vi "Init.vi"(8 "error in (no error)":errorcluster, 11 "Messages Actor in":refnum<class "Messages Actor.lvclass">) -> (0 "error out":errorcluster, 3 "Messages Actor out":refnum<class "Messages Actor.lvclass">)   [LabVIEW 2020, in "Messages Actor.lvlib" / "Messages Actor.lvclass"]
uses:
  Messages Actor.lvclass
  Messages Actor.lvclass/Messages Actor.ctl
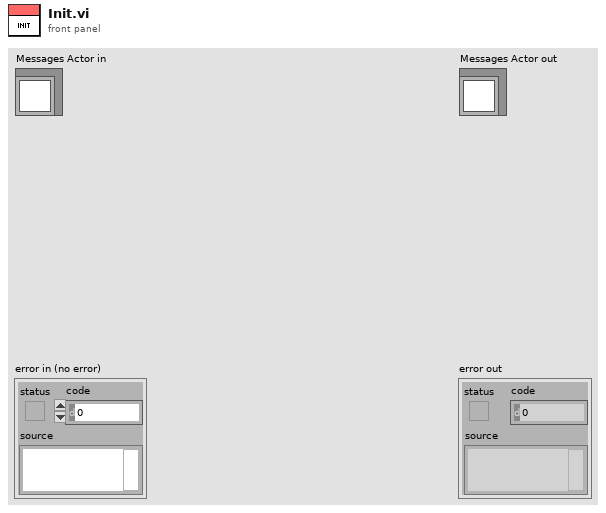
[diagram p1: front panel]
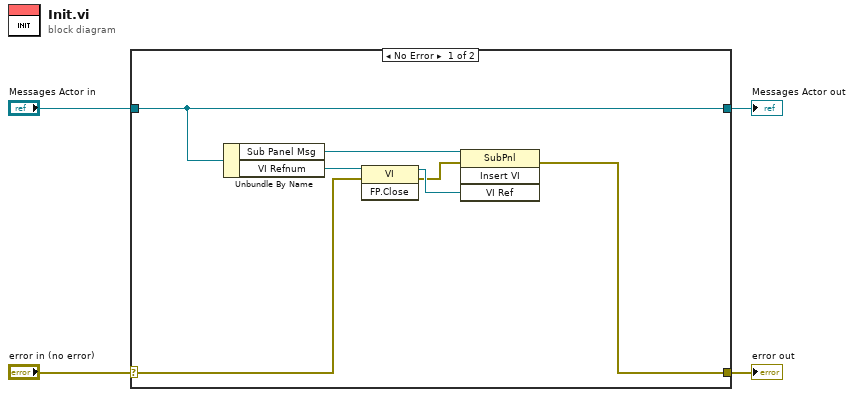
[diagram p0: block diagram]
diagram:
  n1 = case shown="No Error" "error in (no error)" {
    selector: "error in (no error)" -> [w7 w13]
    tunnel: [w6 w13] -> w3
    tunnel: [w5 w12] -> w1
    tunnel: "Messages Actor in" -> [w5 w12]
    frame No Error {
      n2 = Unbundle By Name(w5) -> ("Sub Panel Msg"=w11:refnum<vi>, "VI Refnum"=w10:refnum<vi>)
      n3 = invoke class="VI" method="FP.Close"(reference=w10, error in=w7) -> (reference out=w9:refnum<vi>, error out=w8:errorcluster)  [unwired: 1 in, 1 out]
      n4 = invoke class="SubPnl" method="Insert VI"(reference=w11, error in=w8, "VI Ref"=w9) -> (error out=w6:errorcluster)  [unwired: 1 in, 3 out]
    }
    frame Error {
    }
  }
  "error out" <- w3
  "Messages Actor out" <- w1
